vi "ATF-Pump-ACC_Read.vi"(7 "Data FIFO Ref":T1, 8 "error in (no error)":errorcluster, 9 "number of samples per channel":i32, 10 "ACC_Task":refnum<k21>) -> (0 "error out":errorcluster, 2 "task out":refnum<k21>)   [LabVIEW 2022 SP3]
uses:
  RT Controls/ATF-Pump-Data FIFO.ctl
  <vilib>/Platform/TimedLoop/XDataNode/timing_clust.ctl
  <vilib>/Platform/TimedLoop/XDataNode/nitl_modes.ctl
  <vilib>/Platform/TimedLoop/XDataNode/wakeup.ctl
  <vilib>/DAQmx/read.llb/DAQmx Read (Analog 1D Wfm NChan NSamp).vi
  <vilib>/DAQmx/miscellaneous.llb/DAQmx Fill In Error Info.vi
  <vilib>/platform/TimedLoop/XDataNode/XDataNode.xnode
  <vilib>/Platform/TimedLoop/XDataNode/XDNodeRunTimeDep.lvlib
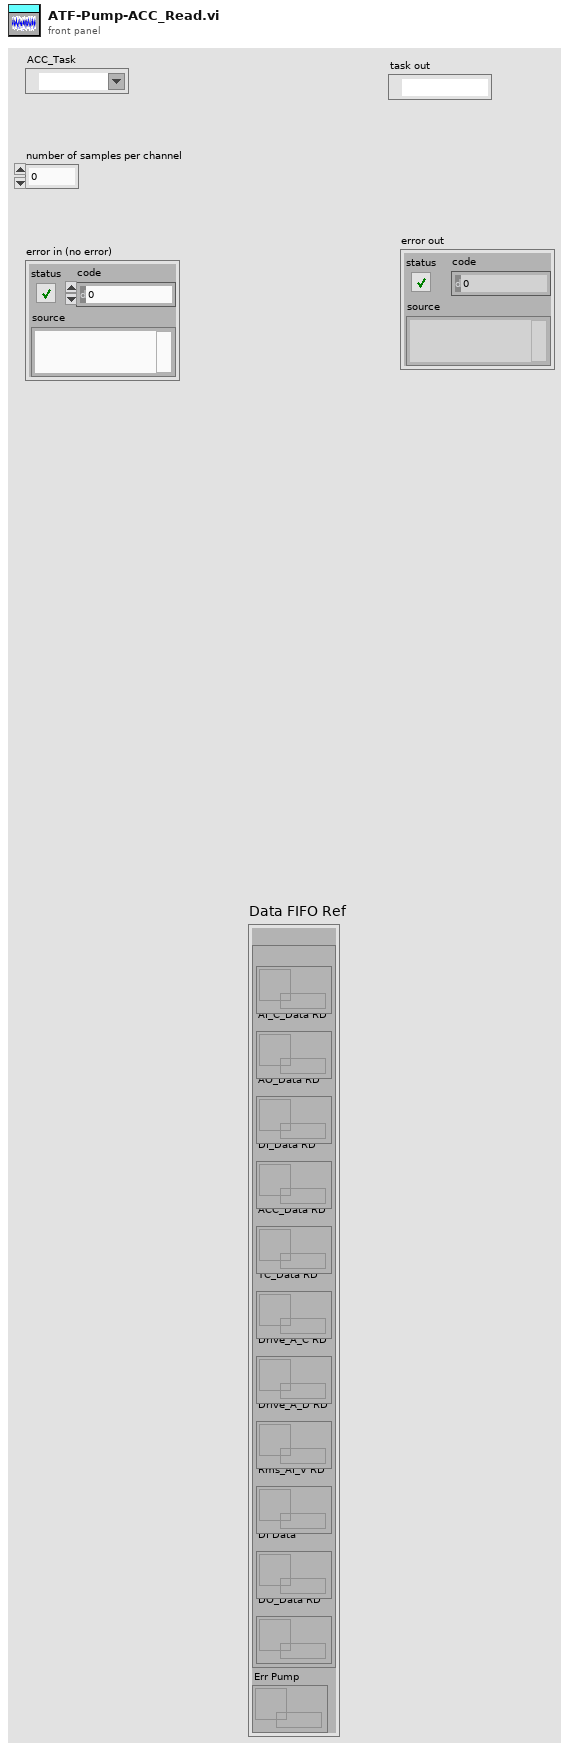
[diagram p1: front panel]
types:
  T1 = typedef "ATF-Pump-Data FIFO.ctl" = cluster{"RD":cluster{"AI_V_Data RD":refnum<queue>, "AI_C_Data RD":refnum<queue>, "AO_Data RD":refnum<queue>, "DI_Data RD":refnum<queue>, "ACC_Data RD":refnum<queue>, "TC_Data RD":refnum<queue>, "Drive_A_C RD":refnum<queue>, "Drive_A_D RD":refnum<queue>, "Rms_AI_V RD":refnum<queue>, "DI Data":refnum<queue>, "DO_Data RD":refnum<queue>}, "Err Pump":refnum<queue>}
  T2 = typedef "XDNodeRunTimeDep.lvlib/timing_clust.ctl" = cluster{"Expected End [f-1]":u64, "Actual End [f-1]":u64, "Finished Late? [f-1]":bool, "Expected End [i-1]":u64, "Actual End [i-1]":u64, "Finished Late? [i-1]":bool, "Expected Start [i]":u64, "Actual Start [i]":u64, "Expected Start [f]":u64, "Actual Start [f]":u64, "Source Name":string, "Structure Name":string, "Period":i64, "Deadline":i64, "Offset":i64, "Start":i64, "Priority":i32, "Timeout":i32, "Mode":T3, "Wakeup Reason":T4, "Error":errorcluster, "Source Type":string, "Secondary Source Type":string, "Global End Time":u64, "Global Start Time":u64, "Frame Duration":u64, "Iteration Duration":u64, "Assigned CPU":i32, "I/O Scan Engine Mode":u32}
  T3 = typedef "XDNodeRunTimeDep.lvlib/nitl_modes.ctl" = enum32{"No Change", "Process missed periods, maintain original phase", "Discard missed periods, maintain original phase", "Process missed periods, ignore original phase", "Discard missed periods, ignore original phase"}
  T4 = typedef "XDNodeRunTimeDep.lvlib/wakeup.ctl" = enum32{"Normal", "Aborted", "Asynchronous wakeup", "Timing source error", "Timed loop error", "Timeout"}
  T5 = enum16{"Init", "Read 'All'", "Read 'n'", "Read '1'", "Write '1'", "Write 'n'", "Write 'All'"}
  T6 = enum16{"AI C", "AI V", "AO", "DI", "DO", "TC", "ACC", "DR L", "DR A"}
  T7 = cluster{"Start DAQ":bool, "Stop DAQ":bool, "RT Stop":bool, "RT Exit":bool, "Start Seq":bool}
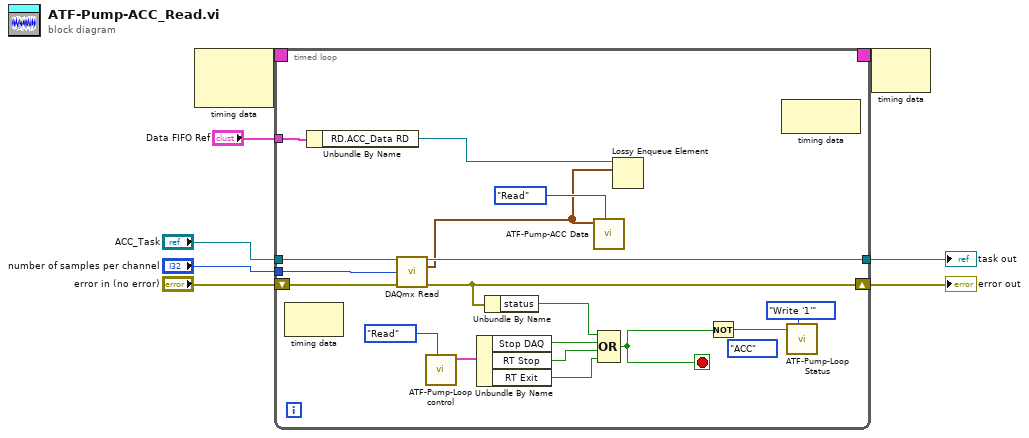
[diagram p0: block diagram]
diagram:
  n1 = node-c288() -> (w8:T2)  [unwired: 2 in]
  n2 = timed-loop {
    shift-right: [w25] -> w2
    shift-left: "error in (no error)" -> [w23]
    tunnel: "ACC_Task" -> [w24]
    tunnel: [w26] -> w5
    tunnel: "number of samples per channel" -> [w22]
    timing: w8 -> [_]
    timing-out: [_] -> w7
    tunnel: "Data FIFO Ref" -> [w14]
    stop <- w10 stop-if-true
    (unwired) T6."ACC" ("Loop")
    n3 = node-c288() -> ()  [unwired: 1 in, 1 out]
    n4 = Unbundle By Name(w14) -> ("RD.ACC_Data RD"=w13:refnum<queue>)
    n5 = call-poly <vilib>:"DAQmx Read.vi"("task/channels in"=w24, "number of samples per channel"=w22, "error in"=w23) -> ("task out"=w26:refnum<k21>, "data"=w12:waveform(dbl)[], "error out"=w25:errorcluster)  [unwired: 10 in]
    n6 = call "ATF-Pump-Loop control.vi"("Action"=enum16{"Init", "Write", "Read"}."Read") -> ("Loop Control out"=w19:T7)  [unwired: 9 in, 1 out]
    n7 = Unbundle By Name(w19) -> ("Stop DAQ"=w18:bool, "RT Stop"=w17:bool, "RT Exit"=w16:bool)
    n8 = Unbundle By Name(w25) -> ("status"=w21:bool)
    n9 = call "ATF-Pump-ACC Data.vi"("Enum"=enum16{"Write", "Read"}."Read", "In_ACC data"=w12) -> ()  [unwired: 9 in, 1 out]
    n10 = Compound Arithmetic op=OR(w21, w18, w17, w16) -> (w10:bool)
    n11 = Lossy Enqueue Element(queue=w13, element=w12) -> ()  [unwired: 1 in, 4 out]
    n12 = Not(x=w10) -> (.not. x?=w11:bool)
    n13 = node-c288() -> ()  [unwired: 1 in, 1 out]
    n14 = call "ATF-Pump-Loop Status.vi"("Option"=T5."Write '1'", "Status"=w11) -> ()  [unwired: 7 in, 3 out]
  }
  "task out" <- w5
  "error out" <- w2
  n15 = node-c288(w7) -> ()  [unwired: 1 out]
